vi "Is Valid File Extension.vi"(8 "error in (no error)":errorcluster, 10 "File extension":string, 11 "Path":path) -> (0 "error out":errorcluster, 1 "Extension of File Found":string, 2 "Is Valid File Extension?":bool)   [LabVIEW 2018, in "Potentiostat Galvanostat.lvclass"]
uses:
  Potentiostat Galvanostat.lvclass
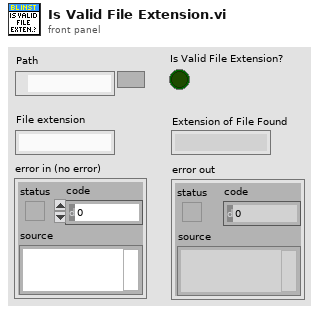
[diagram p1: front panel]
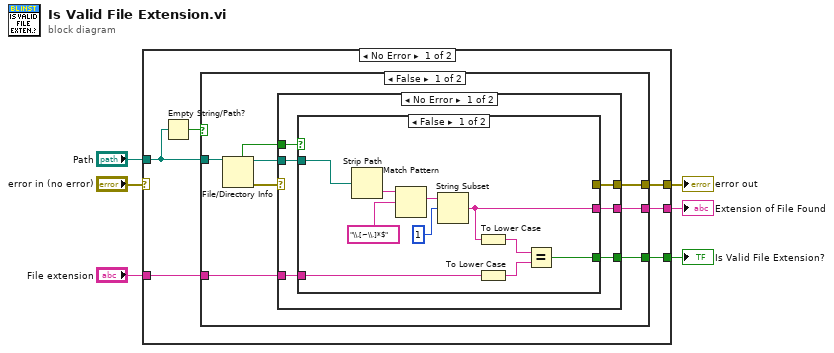
[diagram p0: block diagram]
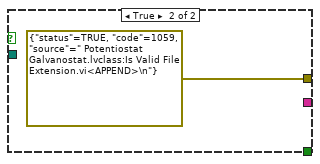
[diagram p2: hidden frame]
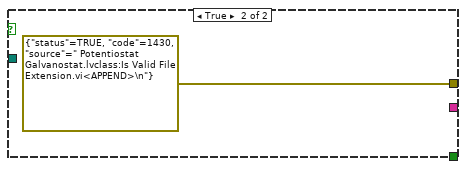
[diagram p4: hidden frame]
diagram:
  n1 = case shown="No Error" "error in (no error)" {
    selector: "error in (no error)" -> [_ w40]
    tunnel: [w12 w40] -> w5
    tunnel: "Path" -> [w11 _]
    tunnel: "File extension" -> [w9 _]
    tunnel: [w8 _] -> w3
    tunnel: [w7 _] -> w2
    frame No Error {
      n2 = Empty String/Path?(string/path=w11) -> (empty?=w10:bool)
      n3 = case shown="False" w10 {
        tunnel: [w20 errorcluster {"status"=TRUE, "code"=1430, "source"=" Potentiostat Galvanostat.lvclass:Is Valid File Extension.vi<APPEND>\n"} ("error out 2")] -> w12
        tunnel: w11 -> [w19 _]
        tunnel: w9 -> [w15 _]
        tunnel: [w14 _] -> w8
        tunnel: [w13 _] -> w7
        frame False {
          n4 = File/Directory Info(path=w19) -> (path out=w18:path, directory=w16:bool, error out=w17:errorcluster)  [unwired: 1 in, 4 out]
          n5 = case shown="No Error" w17 {
            selector: w17 -> [_ w38]
            tunnel: [w24 w38] -> w20
            tunnel: w18 -> [w26 _]
            tunnel: w16 -> [w25 _]
            tunnel: w15 -> [w23 _]
            tunnel: [w22 _] -> w14
            tunnel: [w21 _] -> w13
            frame No Error {
              n6 = case shown="False" w25 {
                tunnel: w26 -> [w34 _]
                tunnel: [_ errorcluster {"status"=TRUE, "code"=1059, "source"=" Potentiostat Galvanostat.lvclass:Is Valid File Extension.vi<APPEND>\n"} ("error out 2")] -> w24
                tunnel: w23 -> [w30 _]
                tunnel: [w31 _] -> w22
                tunnel: [w27 _] -> w21
                frame False {
                  n7 = Strip Path(path=w34) -> (name=w36:string)  [unwired: 1 out]
                  n8 = Match Pattern(string=w36, regular expression="\\.[~\\.]*$") -> (match substring=w33:string)  [unwired: 4 out]
                  n9 = String Subset(string=w33, offset (0)=1) -> (substring=w31:string)  [unwired: 1 out]
                  n10 = To Lower Case(string=w31) -> (all lower case string=w29:string)
                  n11 = To Lower Case(string=w30) -> (all lower case string=w28:string)
                  n12 = Equal?(x=w29, y=w28) -> (x = y?=w27:bool)
                }
                frame True {
                }
              }
            }
            frame Error {
            }
          }
        }
        frame True {
        }
      }
    }
    frame Error {
    }
  }
  "error out" <- w5
  "Extension of File Found" <- w3
  "Is Valid File Extension?" <- w2
